vi "MoveAbs.vi"   [LabVIEW 2019]
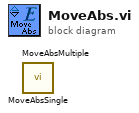
[diagram p0: block diagram]
diagram:
  n1 = call "MoveAbsMultiple.vi"() -> ()  [unwired: 14 in, 2 out]
  n2 = call "MoveAbsSingle.vi"() -> ()  [unwired: 14 in, 2 out]
